vi "ShootWhenReady.vi"(11 "Start Shooting":bool) -> ()   [LabVIEW 2020]
uses:
  <vilib>/Rock Robotics/WPI/ThirdParty/REV Robotics/REVLib/Typedef/Spark MAX Control Type.ctl
  2022 CyberTooth Kokomo/Global Shooter Speed.vi
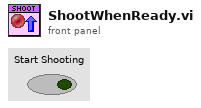
[diagram p1: front panel]
types:
  T1 = typedef "WPI_MotorControlDeviceRef.ctl" = cluster{"DeviceStatus":errorcluster, "Type":T2, "PWM":cluster{"PWM Channel":T3, "DeadBand":T4}, "CAN":cluster{"Device Number":u8, "SetOutput VI Ref":variant, "GetOutput VI Ref":variant, "Enable VI Ref":variant, "Disable VI Ref":variant, "Data":variant}, "Invert":bool, "DIO PWM":cluster{"PWM \"Enable\" Channel":T3, "DIOChannel":T5, "PWM Rate":dbl}}
  T2 = typedef "WPI_MotorControlType.ctl" = enum16{"PWM", "CAN", "DIO PWM"}
  T3 = typedef "FPGA_DIOPWMChannel.ctl" = enum8{"PWM 0", "PWM 1", "PWM 2", "PWM 3", "PWM 4", "PWM 5", "PWM 6", "PWM 7", "PWM 8", "PWM 9", "PWM MXP 0", "PWM MXP 1", "PWM MXP 2", "PWM MXP 3", "PWM MXP 4", "PWM MXP 5", "PWM MXP 6", "PWM MXP 7", "PWM MXP 8", "PWM MXP 9", "Invalid"}
  T4 = typedef "WPI_PWMDeadband.ctl" = cluster{"Name":string, "maxPositivePwm":i32, "minPositivePwm":i32, "centerPwm":i32, "maxNegativePwm":i32, "minNegativePwm":i32, "angularRange":u16}
  T5 = typedef "FPGA_DIOChannel.ctl" = enum8{"DIO 0", "DIO 1", "DIO 2", "DIO 3", "DIO 4", "DIO 5", "DIO 6", "DIO 7", "DIO 8", "DIO 9", "DIO MXP 0", "DIO MXP 1", "DIO MXP 2", "DIO MXP 3", "DIO MXP 4", "DIO MXP 5", "DIO MXP 6", "DIO MXP 7", "DIO MXP 8", "DIO MXP 9", "DIO MXP 10", "DIO MXP 11", "DIO MXP 12", "DIO MXP 13", "DIO MXP 14", "DIO MXP 15", "SPI Port CS1", "SPI Port CS2", "SPI Port CS3", "SPI Port MISO", "SPI Port MOSI", "Invalid"}
  T6 = typedef "WPI_DigitalInputDevRef.ctl" = cluster{"DevStatus":errorcluster, "DIO Channel":T5}
  T7 = typedef "Spark MAX Control Type.ctl" = enum16{"Percent VBus", "Voltage", "Velocity", "Position", "Smart Motion", "Current", "Smart Velocity"}
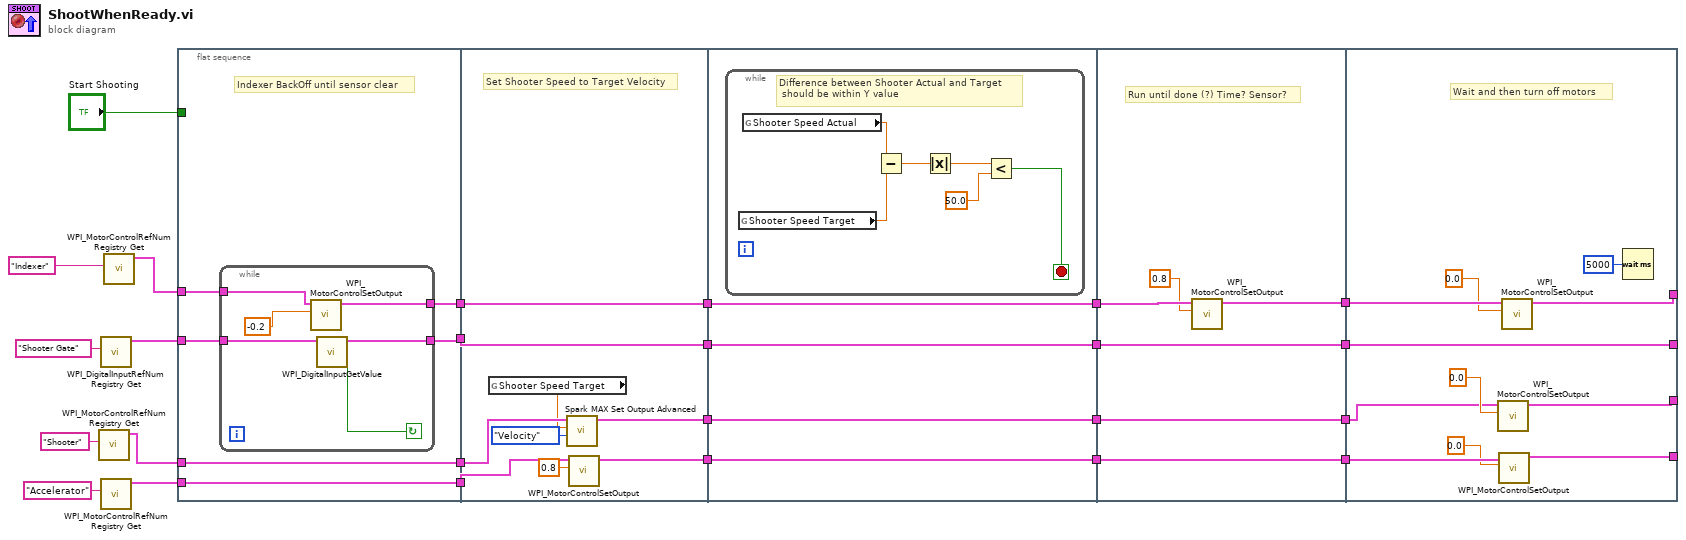
[diagram p0: block diagram]
diagram:
  n1 = call <vilib>:"WPI_MotorControlRefNum Registry Get.vi"("refnum name"="Shooter") -> ("MotorControlDevRef"=w19:T1)  [unwired: 9 in, 1 out]
  n2 = call <vilib>:"WPI_DigitalInputRefNum Registry Get.vi"("refnum name"="Shooter Gate") -> ("DigitalInputDevRef"=w23:T6)  [unwired: 9 in, 1 out]
  n3 = call <vilib>:"WPI_MotorControlRefNum Registry Get.vi"("refnum name"="Accelerator") -> ("MotorControlDevRef"=w15:T1)  [unwired: 9 in, 1 out]
  n4 = call <vilib>:"WPI_MotorControlRefNum Registry Get.vi"("refnum name"="Indexer") -> ("MotorControlDevRef"=w25:T1)  [unwired: 9 in, 1 out]
  n5 = flat-sequence {
    tunnel: w25 -> [w31]
    tunnel: w23 -> [w29]
    tunnel: [w30] -> w21
    tunnel: [w28] -> w20
    tunnel: w19 -> [w27]
    tunnel: [w27] -> w18
    tunnel: w15 -> [w26]
    tunnel: [w26] -> w14
    tunnel: "Start Shooting" -> [_]
    tunnel: w21 -> [w46]
    tunnel: w20 -> [w39]
    tunnel: w18 -> [w43]
    tunnel: w14 -> [w44]
    tunnel: [w46] -> w13
    tunnel: [w42] -> w12
    tunnel: [w45] -> w11
    tunnel: [w39] -> w7
    tunnel: w13 -> [w48]
    tunnel: w12 -> [w50]
    tunnel: w11 -> [w49]
    tunnel: [w50] -> w10
    tunnel: [w49] -> w9
    tunnel: [w48] -> w8
    tunnel: w7 -> [w47]
    tunnel: [w47] -> w6
    tunnel: w10 -> [w62]
    tunnel: w9 -> [w61]
    tunnel: w8 -> [w60]
    tunnel: w6 -> [w57]
    tunnel: [w62] -> w5
    tunnel: [w61] -> w4
    tunnel: [w59] -> w3
    tunnel: [w57] -> w2
    tunnel: w5 -> [w63]
    tunnel: w4 -> [w67]
    tunnel: w3 -> [w72]
    tunnel: [w71] -> _
    tunnel: w2 -> [w69]
    tunnel: [w69] -> _
    tunnel: [w68] -> _
    tunnel: [w66] -> _
    frame #0 {
      # "Indexer BackOff until sensor clear"
      n6 = while {
        tunnel: w31 -> [w37]
        tunnel: [w35] -> w30
        tunnel: w29 -> [w34]
        tunnel: [w33] -> w28
        stop <- w32 continue-if-true
        n7 = call <vilib>:"WPI_MotorControlSetOutput.vi"("Output"=-0.2, "MotorControlDevRef"=w37) -> ("MotorControlDevRef"=w35:T1)  [unwired: 7 in, 2 out]
        n8 = call <vilib>:"WPI_DigitalInputGetValue.vi"("DigitalInputDevRef"=w34) -> ("Value"=w32:bool, "DigitalInputDevRef"=w33:T6)  [unwired: 8 in, 1 out]
      }
    }
    frame #1 {
      # "Set Shooter Speed to Target Velocity"
      n9 = global read "Global Shooter Speed.vi" "Shooter Speed Target"() -> (w41:dbl)
      n10 = call <vilib>:"Spark MAX Set Output Advanced.vi"("Control Mode"=Spark_MAX_Control_Type."Velocity", "Setpoint"=w41, "MotorControlDevRef"=w43) -> ("MotorControlDevRef"=w42:T1)  [unwired: 7 in, 1 out]
      n11 = call <vilib>:"WPI_MotorControlSetOutput.vi"("Output"=0.8, "MotorControlDevRef"=w44) -> ("MotorControlDevRef"=w45:T1)  [unwired: 7 in, 2 out]
    }
    frame #2 {
      n12 = while {
        stop <- w51 stop-if-true
        # "Difference between Shooter Actual and Target\n should be within Y value"
        n13 = global read "Global Shooter Speed.vi" "Shooter Speed Target"() -> (w55:dbl)
        n14 = global read "Global Shooter Speed.vi" "Shooter Speed Actual"() -> (w56:dbl)
        n15 = Subtract(x=w56, y=w55) -> (x-y=w54:dbl)
        n16 = Absolute Value(x=w54) -> (abs(x)=w53:dbl)
        n17 = Less?(x=w53, y=50.0) -> (x < y?=w51:bool)
      }
    }
    frame #3 {
      # "Run until done (?) Time? Sensor?"
      n18 = call <vilib>:"WPI_MotorControlSetOutput.vi"("Output"=0.8, "MotorControlDevRef"=w60) -> ("MotorControlDevRef"=w59:T1)  [unwired: 7 in, 2 out]
    }
    frame #4 {
      # "Wait and then turn off motors"
      n19 = call <vilib>:"WPI_MotorControlSetOutput.vi"("Output"=0.0, "MotorControlDevRef"=w63) -> ("MotorControlDevRef"=w68:T1)  [unwired: 7 in, 2 out]
      n20 = call <vilib>:"WPI_MotorControlSetOutput.vi"("Output"=0.0, "MotorControlDevRef"=w67) -> ("MotorControlDevRef"=w66:T1)  [unwired: 7 in, 2 out]
      n21 = call <vilib>:"WPI_MotorControlSetOutput.vi"("Output"=0.0, "MotorControlDevRef"=w72) -> ("MotorControlDevRef"=w71:T1)  [unwired: 7 in, 2 out]
      n22 = Wait (ms)(milliseconds to wait=u32 5000) -> ()  [unwired: 1 out]
    }
  }
